vi "tester.vi"() -> ()   [LabVIEW 2009]
panel:
  in  "stop":bool
  out "Robot in map":cluster{"Col":dbl, "Row":dbl}
  in  "Walls":cluster{"Col":dbl, "Row":dbl}[](array[cluster])
  in  "Objects bottom cords":T1(array[cluster])
  in  "Robot":cluster{"Col":dbl, "Row":dbl, "Bearing":dbl}
  out "Updated Map":i8[][](array[numeric])
  out "Updated Corners":cluster{"Col":dbl, "Row":dbl}[](array[cluster])
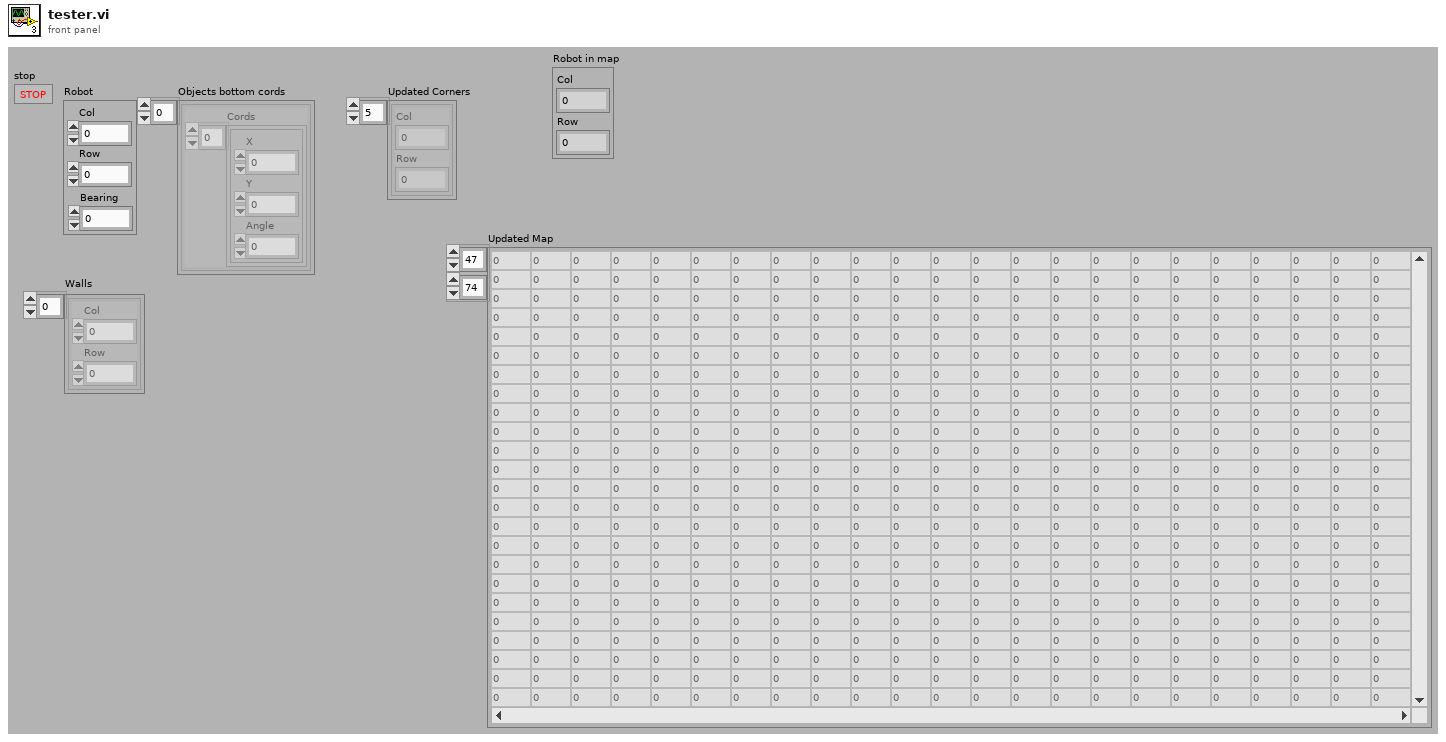
[diagram p1: front panel]
types:
  T1 = cluster{"Cords":cluster{"X":dbl, "Y":dbl, "Angle":dbl}[]}[]
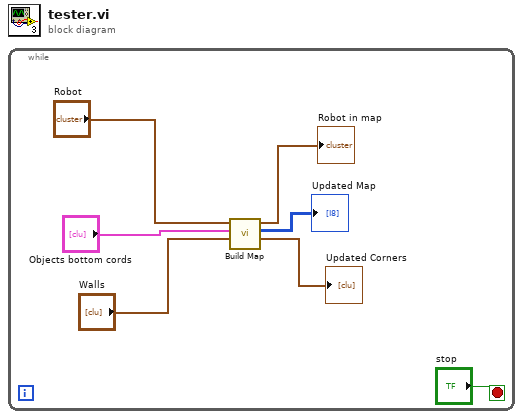
[diagram p0: block diagram]
diagram:
  n1 = while {
    stop <- "stop" stop-if-true
    n2 = call "Build Map.vi"("Walls"="Walls", "Objects bottom cords"="Objects bottom cords", "Robot"="Robot") -> ("Updated Corners"=→"Updated Corners":cluster{"Col":i16, "Row":i16}[], "Updated Map"=→"Updated Map":i8[][], "Robot in map"=→"Robot in map":cluster{"Col":i16, "Row":i16})  [unwired: 2 in]
  }
